vi "Load-from-file-by-reference.vi"(8 "error in (no error)":errorcluster, 9 "Update GUI  values?":bool, 10 "Controls to load":refnum<vi>[](array[refnum]), 11 "Reference in":T2) -> (0 "error out":errorcluster, 2 "Values":T1(array[cluster]), 3 "Reference out":T2)   [LabVIEW 2013, in "SettingsFile.lvlib" / "SettingsFile.lvclass"]
uses:
  SettingsFile.lvclass
  Object-reference.ctl
  Messages.ctl
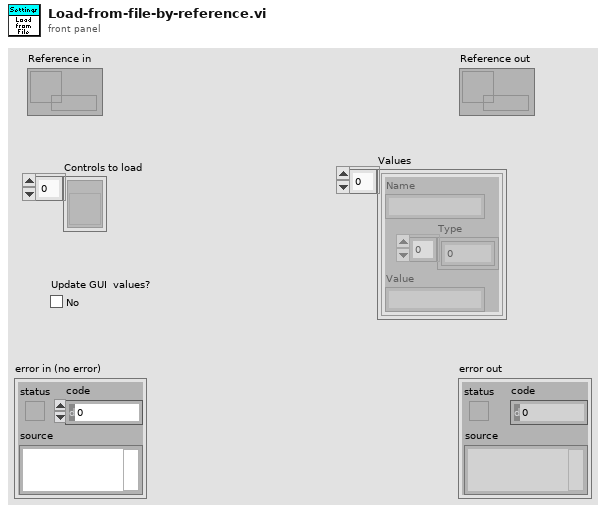
[diagram p1: front panel]
types:
  T1 = cluster{"Name":string, "Type":i16[], "Value":string}[]
  T2 = typedef "SettingsFile.lvlib/SettingsFile.lvclass/Object-reference.ctl" = refnum<data-value>
  T3 = typedef "SettingsFile.lvlib/SettingsFile.lvclass/Messages.ctl" = enum16{"Time out", "User cancel", "Module cancel", "File format change"}
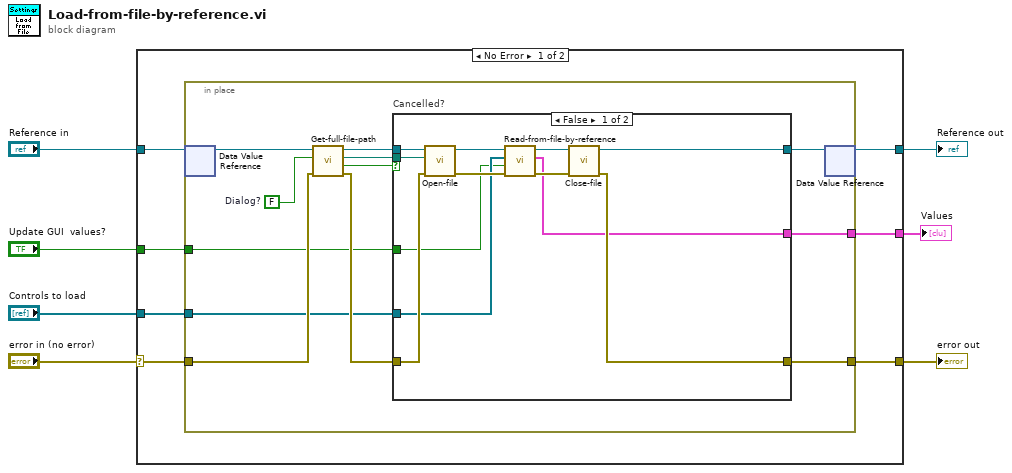
[diagram p0: block diagram]
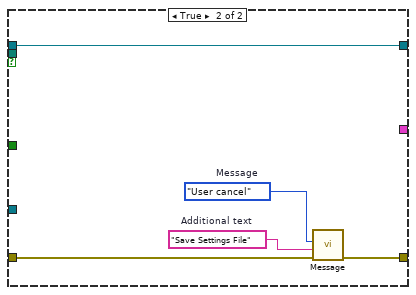
[diagram p2: hidden frame]
diagram:
  n1 = case shown="No Error" "error in (no error)" {
    selector: "error in (no error)" -> [w12 w45]
    tunnel: [w11 w45] -> w6
    tunnel: "Controls to load" -> [w10 _]
    tunnel: "Reference in" -> [w14 w44]
    tunnel: [w13 w44] -> w4
    tunnel: "Update GUI  values?" -> [w9 _]
    tunnel: [w8 _] -> w1
    frame No Error {
      n2 = in-place {
        in-place-border: w12 -> [w21]
        in-place-border: [w19] -> w11
        in-place-border: w10 -> [w17]
        in-place-border: w9 -> [w16]
        in-place-border: [w15] -> w8
        w25 = FALSE  # Dialog?
        n3 = in-place-dvr #1(w14) -> (w26:refnum<class "SettingsFile.lvclass">)  [unwired: 1 out]
        n4 = call "Get-full-file-path.vi"("error in (no error)"=w21, "Dialog?"=w25, "SettingsFile in"=w26) -> ("error out"=w20:errorcluster, "Cancelled?"=w24:bool, "Full path"=w23:path, "SettingsFile out"=w22:refnum<class "SettingsFile.lvclass">)  [unwired: 5 in]
        n5 = case "Cancelled?" shown="False" w24 {
          tunnel: w23 -> [w37 _]
          tunnel: w22 -> [w38 w39]
          tunnel: w20 -> [w32 w43]
          tunnel: [w31 w42] -> w19
          tunnel: w17 -> [w29 _]
          tunnel: [w30 w39] -> w18
          tunnel: w16 -> [w28 _]
          tunnel: [w27 _] -> w15
          frame False {
            n6 = call "Open-file.vi"("error in (no error)"=w32, "Full path"=w37, "SettingsFile in"=w38) -> ("error out"=w35:errorcluster, "SettingsFile out"=w36:refnum<class "SettingsFile.lvclass">)  [unwired: 6 in, 1 out]
            n7 = call "Read-from-file-by-reference.vi"("error in (no error)"=w35, "Update values?"=w28, "Controls by reference"=w29, "SettingsFile in"=w36) -> ("error out"=w33:errorcluster, "Values"=w27:T1, "SettingsFile out"=w34:refnum<class "SettingsFile.lvclass">)  [unwired: 5 in]
            n8 = call "Close-file.vi"("error in (no error)"=w33, "SettingsFile in"=w34) -> ("error out"=w31:errorcluster, "SettingsFile out"=w30:refnum<class "SettingsFile.lvclass">)  [unwired: 8 in]
          }
          frame True {
            w40 = Messages."User cancel"  # Message
            w41 = "Save Settings File"  # Additional text
            n9 = call "Message.vi"("error in (no error)"=w43, "Additional text"=w41, "Message"=w40) -> ("error out"=w42:errorcluster)  [unwired: 8 in]
          }
        }
        n10 = in-place-dvr #1(w18) -> (w13:T2)  [unwired: 1 out]
      }
    }
    frame Error {
    }
  }
  "error out" <- w6
  "Reference out" <- w4
  "Values" <- w1
